vi "Set Debug Mode.vi"(8 "error in (no error)":errorcluster, 10 "Behavior":T1, 11 "SMO":refnum<class "SMO.lvclass">) -> (0 "error out":errorcluster, 3 "SMO out":refnum<class "SMO.lvclass">)   [LabVIEW 2019, in "SMO Debug.lvlib"]
uses:
  SMO Debug.lvlib
  <vilib>/JKI/JKI SMO/SMO/SMO.lvclass
  Attribute.Debug/DebugBehavior.ctl
  Attribute.Debug/Attribute.Debug.lvclass
  SMO.Mediator.lvclass
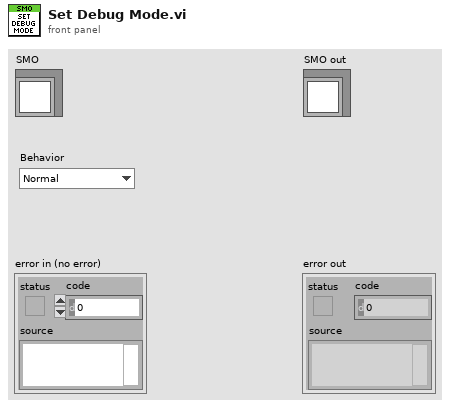
[diagram p1: front panel]
types:
  T1 = typedef "SMO Debug.lvlib/Attribute.Debug.lvclass/DebugBehavior.ctl" = enum16{"Normal", "Debug"}
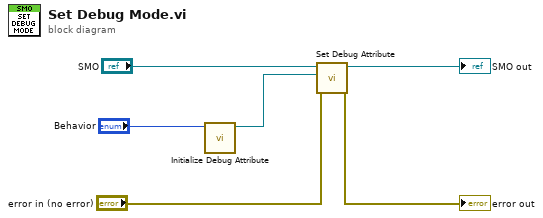
[diagram p0: block diagram]
diagram:
  n1 = call "Initialize Debug Attribute.vi"("Behavior (Normal)"="Behavior") -> ("Attribute.StartupBehavior"=w3:refnum<class "Attribute.Debug.lvclass">)  [unwired: 10 in]
  n2 = call "Set Debug Attribute.vi"("error in (no error)"="error in (no error)", "Attribute.Debug"=w3, "SMO"="SMO") -> ("error out"=→"error out":errorcluster, "SMO out"=→"SMO out":refnum<class "SMO.lvclass">)  [unwired: 7 in]
